vi "test.vi"() -> ()   [LabVIEW 2015]
panel:
  out "Raw data":i32[][][][](array[numeric])
  out "timedelays":dbl[](array[numeric])
  out "waves":dbl[](array[numeric])
  in  "file (use dialog)":path
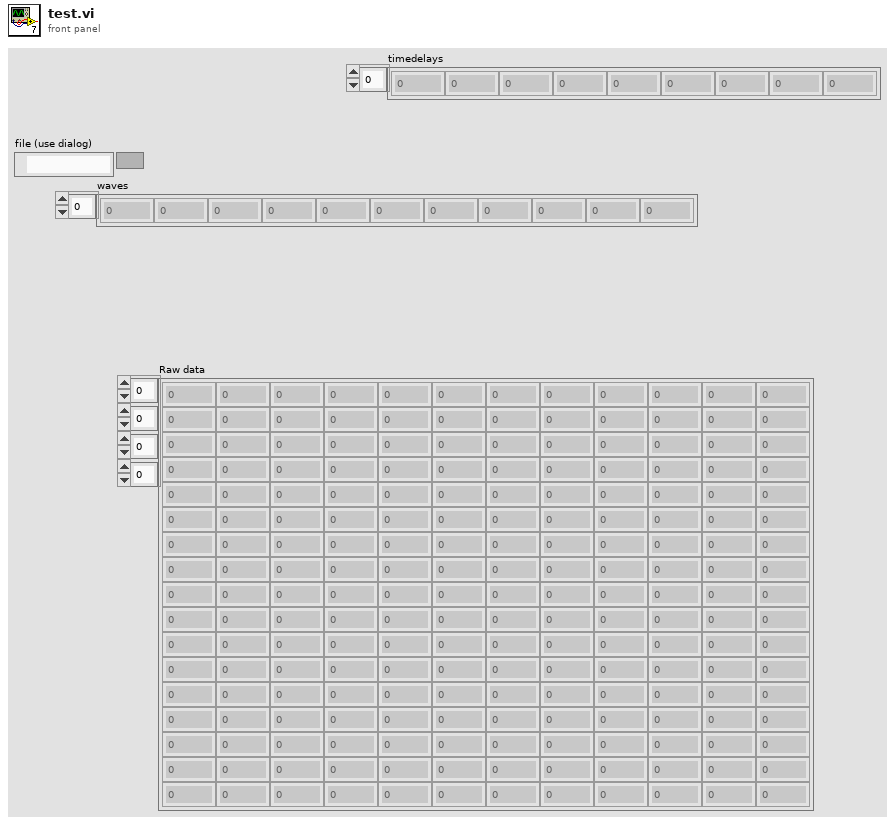
[diagram p1: front panel]
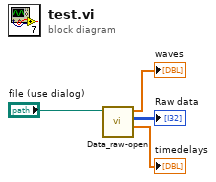
[diagram p0: block diagram]
diagram:
  n1 = call "Data_raw-open.vi"("file (use dialog)"="file (use dialog)") -> ("timedelays"=→"timedelays":dbl[], "Raw data"=→"Raw data":i32[][][][], "waves"=→"waves":dbl[])  [unwired: 8 in]
